vi "Analog FS to mV.vi"(1 "input":i16) -> (0 "output":dbl)   [LabVIEW 2011]
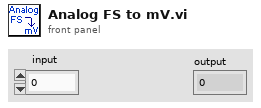
[diagram p1: front panel]
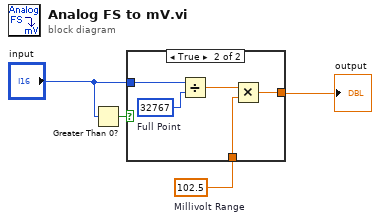
[diagram p0: block diagram]
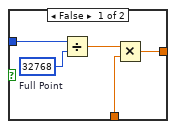
[diagram p2: hidden frame]
diagram:
  w3 = 102.5  # Millivolt Range
  n1 = Greater Than 0?(x="input") -> (x > 0?=w4:bool)
  n2 = case shown="True" w4 {
    tunnel: "input" -> [w6 w14]
    tunnel: [w5 w12] -> w1
    tunnel: w3 -> [w7 w11]
    frame False {
      w8 = 32768  # Full Point
      n3 = Divide(x=w6, y=w8) -> (x/y=w9:dbl)
      n4 = Multiply(x=w9, y=w7) -> (x*y=w5:dbl)
    }
    frame True {
      w10 = 32767  # Full Point
      n5 = Divide(x=w14, y=w10) -> (x/y=w13:dbl)
      n6 = Multiply(x=w13, y=w11) -> (x*y=w12:dbl)
    }
  }
  "output" <- w1
